vi "Start_Serving.vi"() -> ()   [LabVIEW 2015]
doc: "This is a simple example of a server which exports VIs to be called from another machine. You may run both the client.llb and server.llb on the same machine without modifying the access list. If you wish to run the client on another machine that is not in your domain you will have to list the name of the client in the Machine Access List. \n\nThe VIs listed in the Exported VI list are exported by the server.\n\nTo run this example start this VI First, then start the client.llb on all machines you want to try as clients. If you change either of the above lists, you must restart this VI for the changes to take effect.\n\nClick the \"Stop\" button to quit. This will turn off the server, terminating all client connections, and restore the previous access lists to their original values."
uses:
  Anemometry/Anemometry Sub Vis/Globals/Preference_global.vi
panel:
  out "appended path":path
  in  "Srvr.LogEnabled":bool
  out "Exported VI list":string[](array[string])
  # "These are the names of the VIs which will be allowed\nto be accessed from another machine."
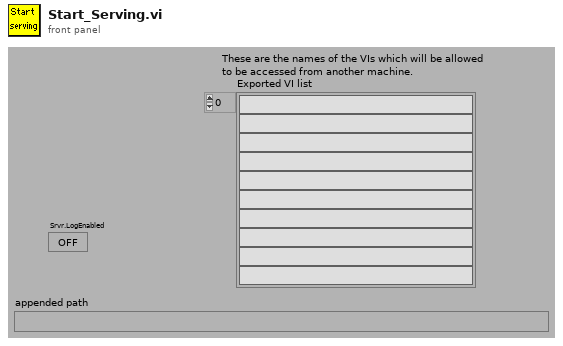
[diagram p1: front panel]
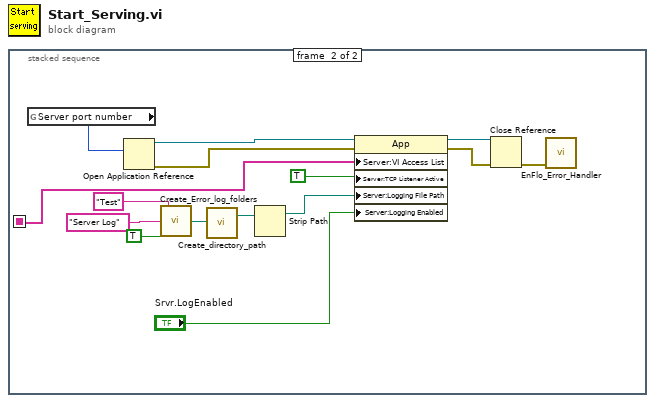
[diagram p0: block diagram]
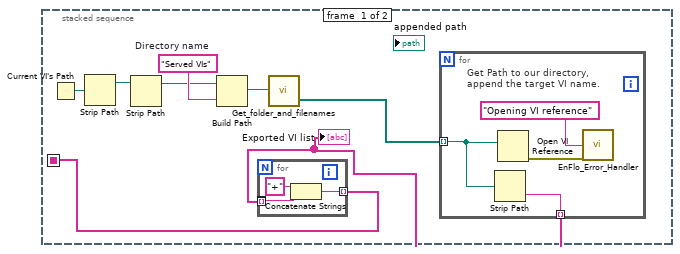
[diagram p2: hidden frame]
diagram:
  n1 = stacked-sequence {
    seq-local: [w6 _] -> [_ w24]
    frame #0 {
      w8 = "Served VIs"  # Directory name
      n2 = Current VI's Path() -> (path=w7:path)
      n3 = Strip Path(path=w7) -> (stripped path=w5:path)  [unwired: 1 out]
      n4 = Strip Path(path=w5) -> (stripped path=w4:path)  [unwired: 1 out]
      n5 = Build Path(base path=w4, name or relative path=w8) -> (appended path=w3:path)
      n6 = call "Get_folder_and_filenames.vi"("file path (dialog if empty)"=w3) -> ("Files"=w2:path[])  [unwired: 1 out]
      n7 = for {
        tunnel: w2 -> [w15] mode=indexing
        tunnel: [w14] -> w1 mode=indexing
        # "Get Path to our directory,\nappend the target VI name."
        n8 = Strip Path(path=w15) -> (name=w14:string)  [unwired: 1 out]
        n9 = Open VI Reference(vi path=w15) -> (error out=w13:errorcluster)  [unwired: 2 in, 4 out]
        n10 = call "EnFlo_Error_Handler.vi"("error in (no error)"=w13, "Error Type"="Opening VI reference") -> ()  [unwired: 1 in, 3 out]
      }
      "Exported VI list" <- w1
      n11 = for {
        tunnel: [w9] -> _ mode=indexing
        tunnel: [w10] -> w6 mode=indexing
        tunnel: w1 -> [w9] mode=indexing
        n12 = Concatenate Strings("+", w9) -> (w10:string)
      }
    }
    frame #1 {
      n13 = global read "Preference_global.vi" "Server port number"() -> (w23:u32)
      n14 = Open Application Reference(10:w23) -> (0:w27:errorcluster, 3:w26:refnum<vi>)  [unwired: 1 in, 2 out]
      n15 = call "Create_Error_log_folders.vi"("Per Day Log File?"=TRUE, "Log Folder"="Server Log", "Log Filename"="Test") -> ("Server copy Location"=w18:path)  [unwired: 2 out]
      n16 = call "Create_directory_path.vi"("Path name"=w18) -> ("Path name Out"=w17:path)  [unwired: 2 in, 1 out]
      n17 = Strip Path(path=w17) -> (stripped path=w19:path)  [unwired: 1 out]
      n18 = property class="App"(reference=w26, error in=w27, "Server:VI Access List"=w24, "Server:TCP Listener Active"=TRUE ("Srvr.TCPActive"), "Server:Logging File Path"=w19, "Server:Logging Enabled"="Srvr.LogEnabled") -> (reference out=w28:refnum<vi>, error out=w29:errorcluster)
      n19 = Close Reference(reference=w28, error in (no error)=w29) -> (error out=w30:errorcluster)
      n20 = call "EnFlo_Error_Handler.vi"("error in (no error)"=w30) -> ()  [unwired: 2 in, 3 out]
    }
  }
